vi "Recieve Request for Result.vi"(6 "Request time":timestamp, 8 "error in (no error)":errorcluster, 9 "Requestor":string, 10 "Requestee":string, 11 "Meter Measurement in":refnum<class "Meter Measurement.lvclass">) -> (0 "error out":errorcluster, 3 "Meter Measurement out":refnum<class "Meter Measurement.lvclass">)   [LabVIEW 2015, in "Meter Measurement.lvclass"]
uses:
  Meter Measurement.lvclass
  Mag Lab Root/Mag Lab Root.lvclass/Mag Lab Root.ctl
  <vilib>/ActorFramework/Actor/Actor.lvclass/Actor.ctl
  Meter Measurement.lvclass/Meter Measurement.ctl
  Mag Lab Root Messages/Recieve Request for Result Msg/Recieve Request for Result Msg.lvclass/Recieve Request for Result Msg.ctl
  <vilib>/ActorFramework/Message Enqueuer/Message Enqueuer.lvclass/Message Enqueuer.ctl
  <vilib>/ActorFramework/Message Enqueuer/Enqueue.vi
  <vilib>/ActorFramework/Message Priority Queue/Priority Enqueue.vi
  Mag Lab Root Messages/Recieve Request for Result Msg/Recieve Request for Result Msg.lvclass
  <vilib>/ActorFramework/Actor/Actor.lvclass
  Mag Lab Error Handler/Mag Lab Error Handler.lvclass
  Mag Lab Root/Mag Lab Root.lvclass
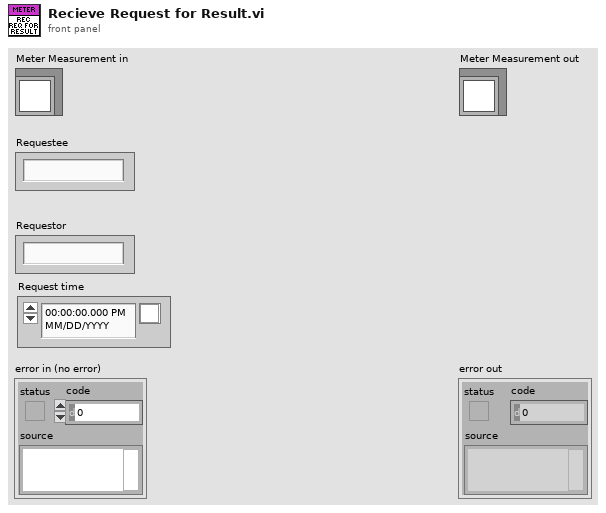
[diagram p1: front panel]
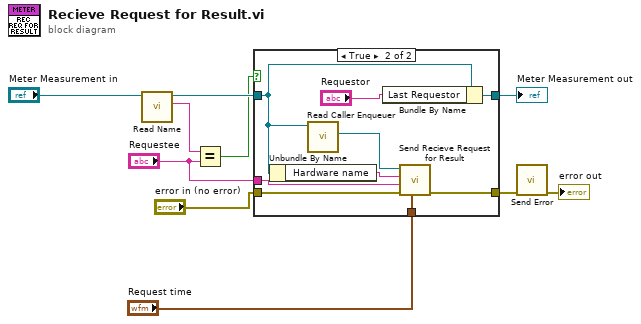
[diagram p0: block diagram]
diagram:
  n1 = call "Read Name.vi"("Mag Lab Root in"="Meter Measurement in") -> ("Name"=w3:string, "Mag Lab Root out"=w5:refnum<class "Meter Measurement.lvclass">)  [unwired: 8 in, 1 out]
  n2 = Equal?(x=w3, y="Requestee") -> (x = y?=w4:bool)
  n3 = case shown="True" w4 {
    tunnel: "error in (no error)" -> [w11 w19]
    tunnel: [w11 w18] -> w8
    tunnel: [w12 w17] -> w7
    tunnel: w5 -> [w12 w15]
    tunnel: "Requestee" -> [_ w14]
    tunnel: "Request time" -> [_ w13]
    frame False {
    }
    frame True {
      n4 = Unbundle By Name(w15) -> ("Hardware name"=w20:string)
      n5 = call <vilib>:"Read Caller Enqueuer.vi"("Actor"=w15) -> ("Caller Enqueuer"=w21:refnum<class "Message Enqueuer.lvclass">)  [unwired: 10 in]
      n6 = Bundle By Name(cluster=w15, "Last Requestor"="Requestor") -> (w17:refnum<class "Meter Measurement.lvclass">)
      n7 = call "Send Recieve Request for Result.vi"("Request time"=w13, "error in (no error)"=w19, "Requestor"=w14, "Requestee"=w20, "Message Enqueuer"=w21) -> ("error out"=w18:errorcluster)  [unwired: 5 in, 1 out]
    }
  }
  "Meter Measurement out" <- w7
  n8 = call "Send Error.vi"("error in (no error)"=w8) -> ("error out"=→"error out":errorcluster)  [unwired: 9 in, 1 out]
